vi "Write Test Case.vi"(10 "Test Case":string, 11 "Method Result In":refnum<class "Method Result.lvclass">) -> (3 "Method Result Out":refnum<class "Method Result.lvclass">)   [LabVIEW 2020, in "Method Result.lvclass"]
uses:
  Method Result.lvclass
  Method Result.lvclass/Method Result.ctl
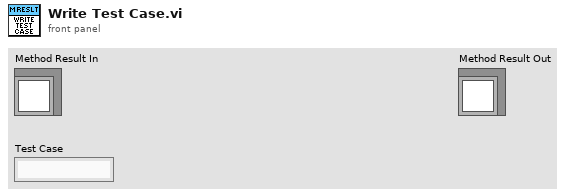
[diagram p1: front panel]
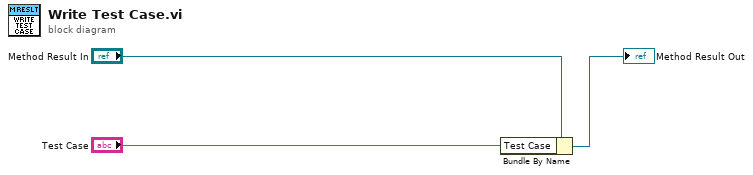
[diagram p0: block diagram]
diagram:
  n1 = Bundle By Name(cluster="Method Result In", "Test Case"="Test Case") -> (→"Method Result Out":refnum<class "Method Result.lvclass">)
